vi "ReadVision.vi"(3 "Name":string="Pixy") -> (1 "Target Data":u16[](array[numeric]))   [LabVIEW 2016]
doc: "ADXL362 SPI Accelerometer\n\nThis example shows how to use the Analog Devices ADXL362 Accelerometer sensor connected to SPI.\n\nThis example expects a USB cable connected from your development PC to the Type B USB Jack (next to the power input) on the roboRIO."
panel:
  in  "Max Bytes To Read":u8=100
  out "Checksum":u16
  out "Bytes Read":u16
  out "Read Zeros":bool
  out "out of sync":bool
  out "CC Block":bool
  out "All Data":u16[](array[numeric])
  out "error out":errorcluster
  # "Set these inputs before running."
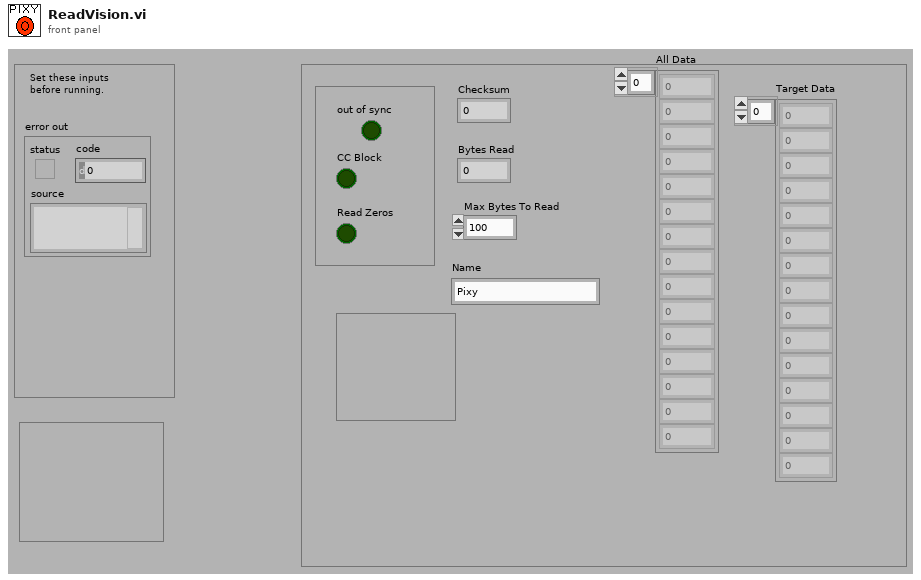
[diagram p1: front panel]
types:
  T1 = typedef "WPI_I2CDevRef.ctl" = cluster{"DevStatus":errorcluster, "Device Address":u8, "Handle":i32, "I2C Bus":T2}
  T2 = typedef "i2c_bus.ctl" = enum16{"I2C On-Board", "I2C MXP", "Invalid"}
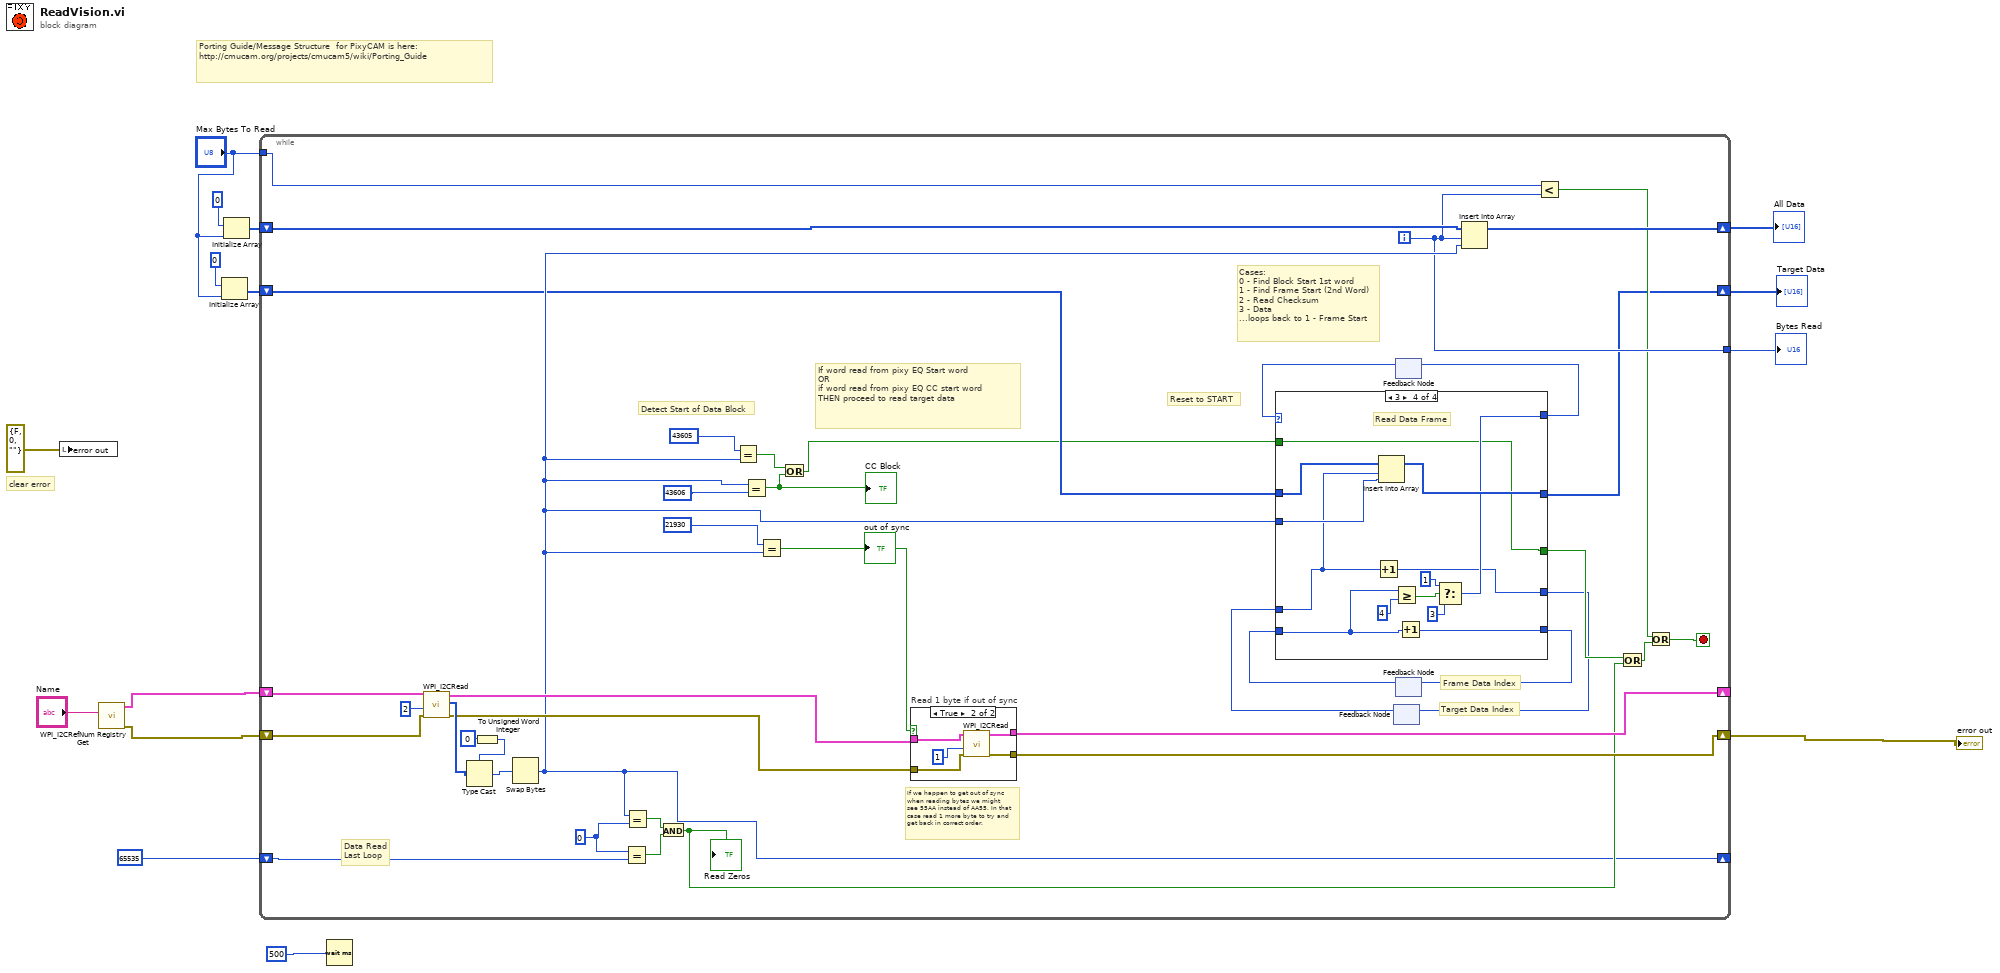
[diagram p0: block diagram]
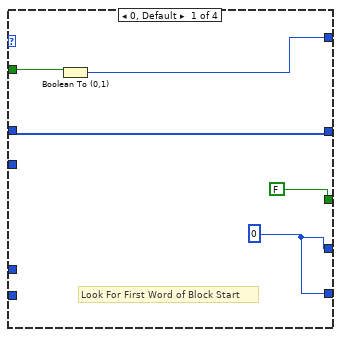
[diagram p2: hidden frame]
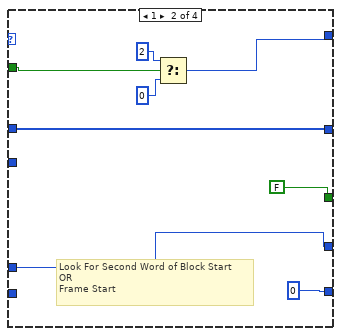
[diagram p3: hidden frame]
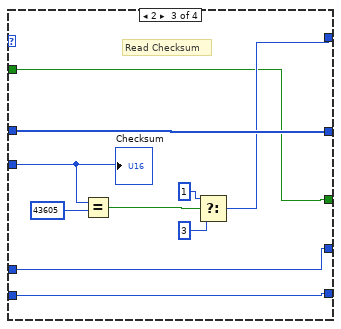
[diagram p4: hidden frame]
diagram:
  # "Porting Guide/Message Structure  for PixyCAM is here:\nhttp://cmucam.org/projects/cmucam5/wiki/Porting_Guide"
  # "clear error"
  n1 = local write "error out"(errorcluster {"status"=FALSE, "code"=0, "source"=""} ("error out")) -> ()
  n2 = call <vilib>:"WPI_I2CRefNum Registry Get.vi"("refnum name"="Name") -> ("error out"=w2:errorcluster, "I2CDevRef"=w3:T1)  [unwired: 9 in]
  n3 = Initialize Array(0, "Max Bytes To Read") -> (w6:i32[])
  n4 = Initialize Array(0, "Max Bytes To Read") -> (w10:i32[])
  n5 = while {
    shift-right: [w48] -> w14
    shift-left: w2 -> [w18]
    shift-right: [w49] -> _
    shift-left: w3 -> [w42]
    shift-right: [w55] -> w11
    shift-left: w10 -> [w32]
    shift-right: [w33] -> _
    shift-left: u16 65535 -> [w30]
    tunnel: [w29] -> w8
    tunnel: "Max Bytes To Read" -> [w34]
    shift-right: [w17] -> w5
    shift-left: w6 -> [w31]
    i -> [w29]
    stop <- w26 stop-if-true
    w37 = u16 0
    # "If word read from pixy EQ Start word\nOR\nif word read from pixy EQ CC start word\nTHEN proceed to read target data"
    # "Cases:\n0 - Find Block Start 1st word\n1 - Find Frame Start (2nd Word)\n2 - Read Checksum\n3 - Data\n...loops back to 1 - Frame Start"
    # "Target Data Index"
    # "Frame Data Index"
    # "Data Read\nLast Loop"
    # "Reset to START"
    # "If we happen to get out of sync\nwhen reading bytes we might\nsee 55AA instead of AA55. In that\ncase read 1 more byte to try and\nget back in correct order."
    # "Detect Start of Data Block"
    n6 = call <vilib>:"WPI_I2CRead.vi"("error in (no error)"=w18, "I2CBytesToRead"=u8 2, "I2CDevRef"=w42) -> ("error out"=w36:errorcluster, "Data Out"=w44:u8[], "I2CDevRef"=w41:T1)  [unwired: 6 in]
    n7 = To Unsigned Word Integer(number=0 ("type")) -> (unsigned 16bit integer=w45:u16)
    n8 = Type Cast(type=w45, x=w44) -> (*(type *) &x=w43:u16)
    n9 = Swap Bytes(anything=w43) -> (byte swapped=w33:u16)
    n10 = Equal?(x=w37, y=w30) -> (x = y?=w51:bool)
    n11 = Equal?(x=w33, y=w37) -> (x = y?=w52:bool)
    n12 = And(x=w52, y=w51) -> (x .and. y?=w35:bool)
    "Read Zeros" <- w35
    n13 = Equal?(x=u16 43605, y=w33) -> (x = y?=w54:bool)
    n14 = Equal?(x=w33, y=u16 43606) -> (x = y?=w50:bool)
    "CC Block" <- w50
    n15 = Equal?(x=u16 21930, y=w33) -> (x = y?=w53:bool)
    "out of sync" <- w53
    n16 = Or(x=w54, y=w50) -> (x .or. y?=w22:bool)
    n17 = case "Read 1 byte if out of sync" shown="True" w53 {
      tunnel: w41 -> [w93 w98]
      tunnel: [w93 w97] -> w49
      tunnel: [w92 w95] -> w48
      tunnel: w36 -> [w92 w94]
      frame False {
        # "If not out of sync\nthen do nothing"
      }
      frame True {
        n18 = call <vilib>:"WPI_I2CRead.vi"("error in (no error)"=w94, "I2CBytesToRead"=u8 1, "I2CDevRef"=w98) -> ("error out"=w95:errorcluster, "I2CDevRef"=w97:T1)  [unwired: 6 in, 1 out]
      }
    }
    n19 = feedback #1() -> (w19:i32)  [unwired: 1 in]
    n20 = feedback #2() -> (w27:i32)  [unwired: 1 in]
    n21 = feedback #3() -> (w21:i32)  [unwired: 1 in]
    n22 = case shown="3" w27 {
      tunnel: w33 -> [_ _ w76 w90]
      tunnel: w31 -> [w60 w68 w78 w80]
      tunnel: [w60 w68 w78 w91] -> w17
      tunnel: [w56 0 w70 w83] -> w16
      tunnel: w22 -> [w59 w61 w71 w85]
      tunnel: [w58 w64 w72 w87] -> w28
      tunnel: [FALSE FALSE w71 w85] -> w23
      tunnel: w21 -> [_ _ w70 w82]
      tunnel: w19 -> [_ w62 w69 w79]
      tunnel: [w56 w62 w69 w81] -> w20
      frame 0, Default {
        w56 = 0
        # "Look For First Word of Block Start"
        n23 = Boolean To (0,1)(Boolean=w59) -> (0, 1=w58:i16)
      }
      frame 1 {
        # "Look For Second Word of Block Start\nOR\nFrame Start"
        n24 = Select(t=2, s=w61, f=0) -> (s? t:f=w64:i32)
      }
      frame 2 {
        # "Read Checksum"
        n25 = Equal?(x=w76, y=u16 43605) -> (x = y?=w75:bool)
        n26 = Select(t=1, s=w75, f=3) -> (s? t:f=w72:i32)
        "Checksum" <- w76
      }
      frame 3 {
        # "Read Data Frame"
        n27 = Increment(x=w79) -> (x+1=w81:i32)
        n28 = Insert Into Array(array=w80, index=w79, new element=w90) -> (w91:i32[])
        n29 = Greater Or Equal?(x=w82, y=4) -> (x >= y?=w84:bool)
        n30 = Increment(x=w82) -> (x+1=w83:i32)
        n31 = Select(t=1, s=w84, f=3) -> (s? t:f=w87:i32)
      }
    }
    n32 = feedback-in #1(w20) -> ()
    n33 = feedback-in #2(w28) -> ()
    n34 = feedback-in #3(w16) -> ()
    n35 = Insert Into Array(array=w32, index=w29, new element=w33) -> (w55:i32[])
    n36 = Less?(x=w34, y=w29) -> (x < y?=w25:bool)
    n37 = Or(x=w23, y=w35) -> (x .or. y?=w24:bool)
    n38 = Or(x=w25, y=w24) -> (x .or. y?=w26:bool)
  }
  "error out" <- w14
  "All Data" <- w11
  "Bytes Read" <- w8
  "Target Data" <- w5
  n39 = Wait (ms)(milliseconds to wait=500) -> ()  [unwired: 1 out]
